vi "SetdBAux.vi"(8 "错误输入（无错误）":errorcluster, 10 "辅助增益值":u16) -> (0 "错误输出":errorcluster)   [LabVIEW 2014]
uses:
  X86Dll/ZXUTConfigMgr.dll
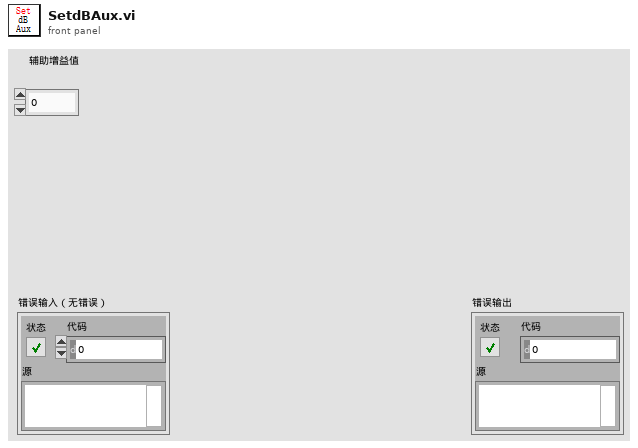
[diagram p1: front panel]
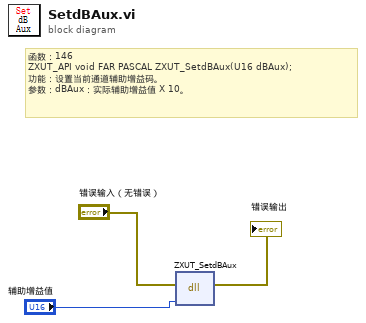
[diagram p0: block diagram]
diagram:
  # "函数：146\nZXUT_API void\tFAR PASCAL ZXUT_SetdBAux(U16 dBAux);\n功能：设置当前通道辅助增益码。\n参数：dBAux：实际辅助增益值 X 10。"
  n1 = dll-call lib="D:/Software/Utrasonic on-line monitoring/X86Dll/ZXUTConfigMgr.dll" fn="ZXUT_SetdBAux"(error in="错误输入（无错误）", "dBAux"="辅助增益值") -> (error out=→"错误输出":errorcluster)  [unwired: 4 in, 1 out]
